vi "Read Nested Queues.vi"(8 "error in (no error)":errorcluster, 11 "Generic Actor in":refnum<class "Generic Actor.lvclass">) -> (0 "error out":errorcluster, 2 "Nested Enqueues":refnum<class "Message Enqueuer.lvclass">[](array[class]), 3 "Generic Actor out":refnum<class "Generic Actor.lvclass">)   [LabVIEW 2020, in "Generic Actor.lvlib" / "Generic Actor.lvclass"]
uses:
  Generic Actor.lvclass
  <vilib>/ActorFramework/Message Enqueuer/Message Enqueuer.lvclass
  Generic Actor.lvclass/Generic Actor.ctl
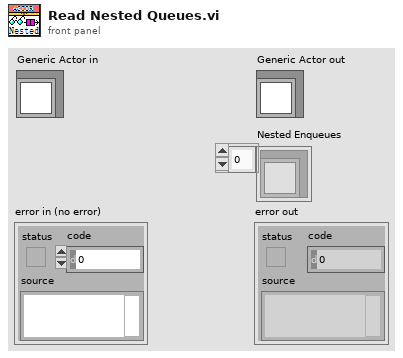
[diagram p1: front panel]
types:
  T1 = map{string, refnum<class "Message Enqueuer.lvclass">}
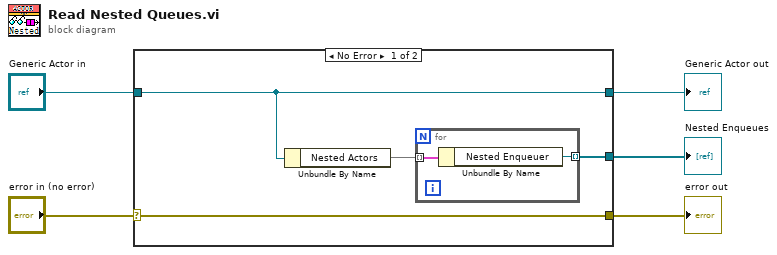
[diagram p0: block diagram]
diagram:
  n1 = case shown="No Error" "error in (no error)" {
    selector: "error in (no error)" -> [w9 w13]
    tunnel: [w9 w13] -> w4
    tunnel: [w8 w12] -> w2
    tunnel: "Generic Actor in" -> [w8 w12]
    tunnel: [w6 _] -> w1
    frame No Error {
      n2 = Unbundle By Name(w8) -> ("Nested Actors"=w7:T1)
      n3 = for {
        tunnel: w7 -> [w11] mode=indexing
        tunnel: [w10] -> w6 mode=indexing
        n4 = Unbundle By Name(w11) -> ("Nested Enqueuer"=w10:refnum<class "Message Enqueuer.lvclass">)
      }
    }
    frame Error {
    }
  }
  "error out" <- w4
  "Generic Actor out" <- w2
  "Nested Enqueues" <- w1
